vi "FFT_example.vi"() -> ()   [LabVIEW 2013]
uses:
  <vilib>/Analysis/2dsp.llb/Real FFT.vi
  <vilib>/Utility/file.llb/Read From Spreadsheet File (DBL).vi
  <vilib>/Analysis/NI_AALPro.lvlib
panel:
  out "LINE SPREAD FUNCTION":dbl[](graph)
  out "ESF":dbl[](graph)
  out "dimensione(X)":dbl
  out "MTF":dbl[](graph)
  out "abs(x)":dbl[](array[numeric])
  out "FFT {X}":cdb[](array[numeric])=[34.0+0.0i, -30.85207104105635-2.4281106500055203i, 23.44988535740028+3.7140969680063827i, -15.677638464676523-3.7638679879062367i, 9.634800400218285+3.1305364193036116i, -5.124873734152915-2.122792206135786i, 1.7043718084221333+0.868420811791921i, 0.3758175248044425+0.2303012753969622i, -1.080369543531189-0.7849344193371482i, 1.0613031914214286+0.906438557213779i, -0.8999999999999986-0.8999999999999986i, 0.64248658531159+0.7522551396452025i, -0.25980040021828493-0.3575845737916235i, -0.0452775464219288-0.07388624051767707i, 0.15069850070388524+0.29576246064532213i, -0.17512626584708346-0.4227922061357852i, 0.20536954353118964+0.6320624631631395i, -0.1828941823316309-0.7618090956168174i, 0.09504433347370028+0.6000863044308599i, -0.021726067051022525-0.276055856062162i, 0.0+0.0i, -0.021726067051022525+0.276055856062162i, 0.09504433347370028-0.6000863044308599i, -0.1828941823316309+0.7618090956168174i, 0.20536954353118964-0.6320624631631395i, -0.17512626584708346+0.4227922061357852i, 0.15069850070388524-0.29576246064532213i, -0.0452775464219288+0.07388624051767707i, -0.25980040021828493+0.3575845737916235i, 0.64248658531159-0.7522551396452025i, -0.8999999999999986+0.8999999999999986i, 1.0613031914214286-0.906438557213779i, -1.080369543531189+0.7849344193371482i, 0.3758175248044425-0.2303012753969622i, 1.7043718084221333-0.868420811791921i, -5.124873734152915+2.122792206135786i, 9.634800400218285-3.1305364193036116i, -15.677638464676523+3.7638679879062367i, 23.44988535740028-3.7140969680063827i, -30.85207104105635+2.4281106500055203i]
  in  "X":dbl[](array[numeric])=[0.0, 0.0, 0.0, 0.0, 0.0, 0.0, 0.0, 0.0, 0.0, 0.0, 0.1, 0.15, 0.2, 0.3, 0.45, 0.9, 1.8, 3.6, 4.5, 5.0, 5.0, 4.5, 3.6, 1.8, 0.9, 0.45, 0.3, 0.2, 0.15, 0.1, 0.0, 0.0, 0.0, 0.0, 0.0, 0.0, 0.0, 0.0, 0.0, 0.0]
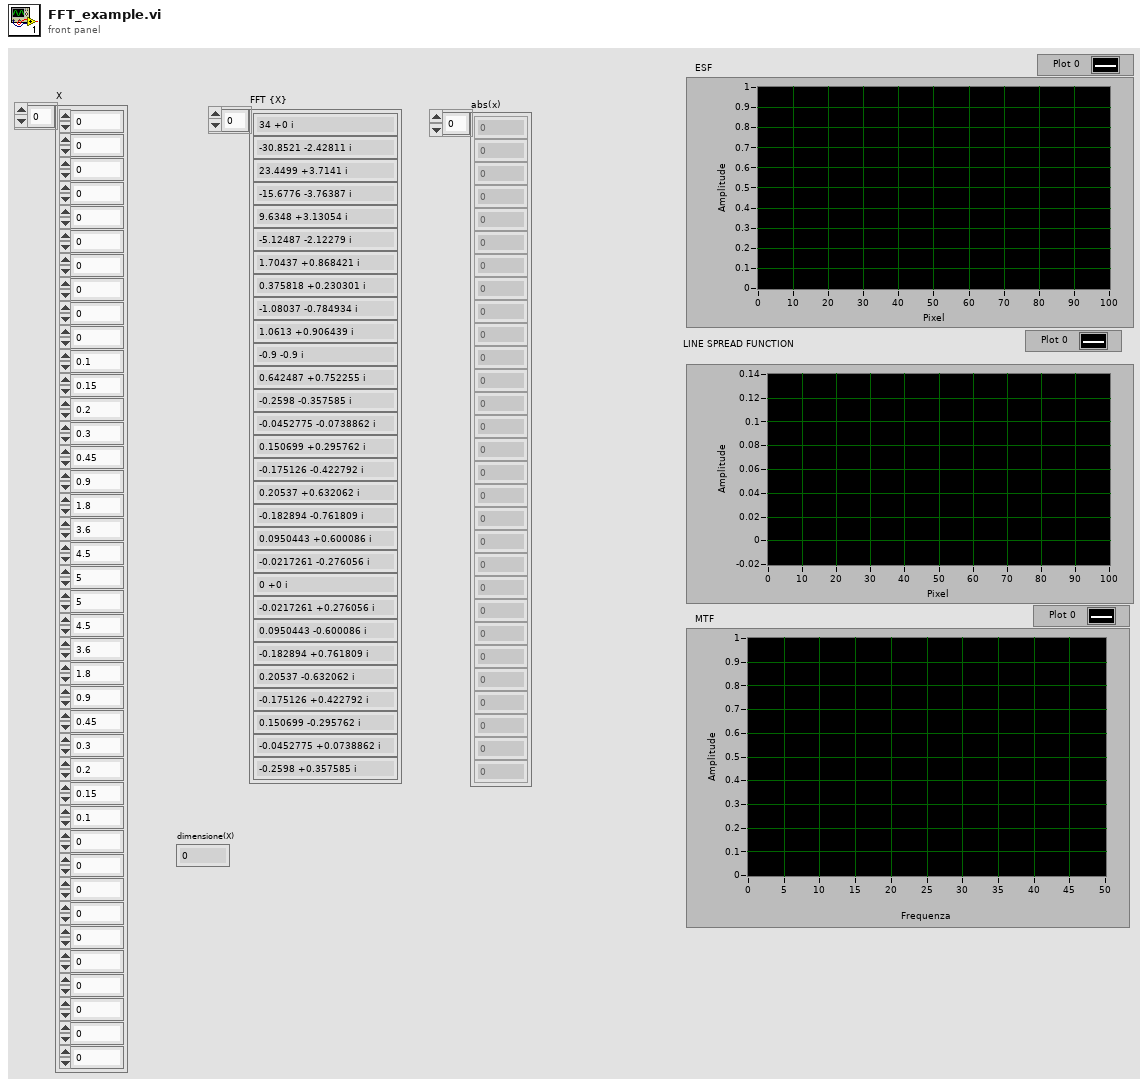
[diagram p1: front panel]
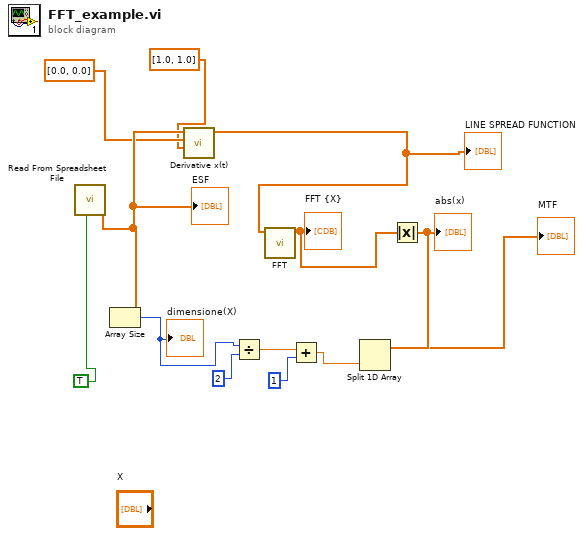
[diagram p0: block diagram]
diagram:
  n1 = call-poly <vilib>:"Read From Spreadsheet File.vi"("transpose (no:F)"=TRUE) -> ("first row"=w4:dbl[])  [unwired: 6 in, 4 out]
  "ESF" <- w4
  n2 = Array Size(array=w4) -> (size(s)=w10:i32)
  "dimensione(X)" <- w10
  n3 = call <vilib>:"Derivative x(t).vi"("Final Condition"=dbl[] [1.0, 1.0], "Initial Condition"=dbl[] [0.0, 0.0], "X"=w4) -> ("dX/dt"=w3:dbl[])  [unwired: 7 in, 1 out]
  "LINE SPREAD FUNCTION" <- w3
  n4 = Divide(x=w10, y=2) -> (x/y=w9:dbl)
  n5 = call-poly <vilib>:"FFT.vi"("X"=w3) -> ("FFT {X}"=w13:cdb[])  [unwired: 9 in, 1 out]
  "FFT {X}" <- w13
  n6 = Add(x=w9, y=1) -> (x+y=w8:dbl)
  n7 = Absolute Value(x=w13) -> (abs(x)=w7:dbl[])
  "abs(x)" <- w7
  n8 = Split 1D Array(array=w7, index=w8) -> (first subarray=→"MTF":dbl[])  [unwired: 1 out]
